vi "Tic Tac Toe.vi"() -> ()   [LabVIEW 2015]
panel:
  out "String 7":string="TIC TAC TOE GAME"
  in  "Tab Control":enum32{"Page 1", "Page 2"}(tab)
  in  "OK Button 9":bool
  in  "OK Button 8":bool
  in  "OK Button 7":bool
  in  "OK Button 6":bool
  in  "OK Button 5":bool
  in  "OK Button 4":bool
  in  "OK Button 3":bool
  in  "OK Button 2":bool
  in  "OK Button":bool
  in  "Text Colour X":u32(colorbox)
  in  "Text Colour O":u32(colorbox)
  in  "OK Button 12":bool
  in  "OK Button 11":bool
  out "Next Turn":string
  in  "OK Button 10":bool
  out "String 2":string="Player 1"
  out "String":string="Player 2"
  in  "Set Player Turn":bool
  out "String 6":string="O"
  out "String 5":string="X"
  out "String 10":string
  out "x .and. y?":bool
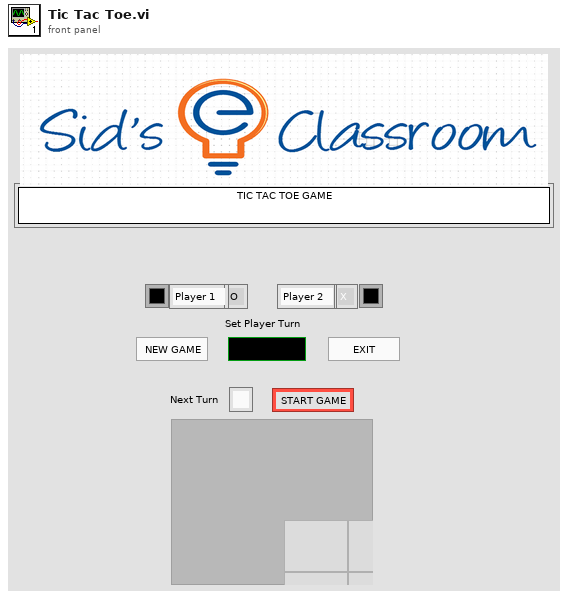
[diagram p1: front panel]
types:
  T1 = enum8{"Enabled", "Disabled", "Disabled and Grayed Out"}
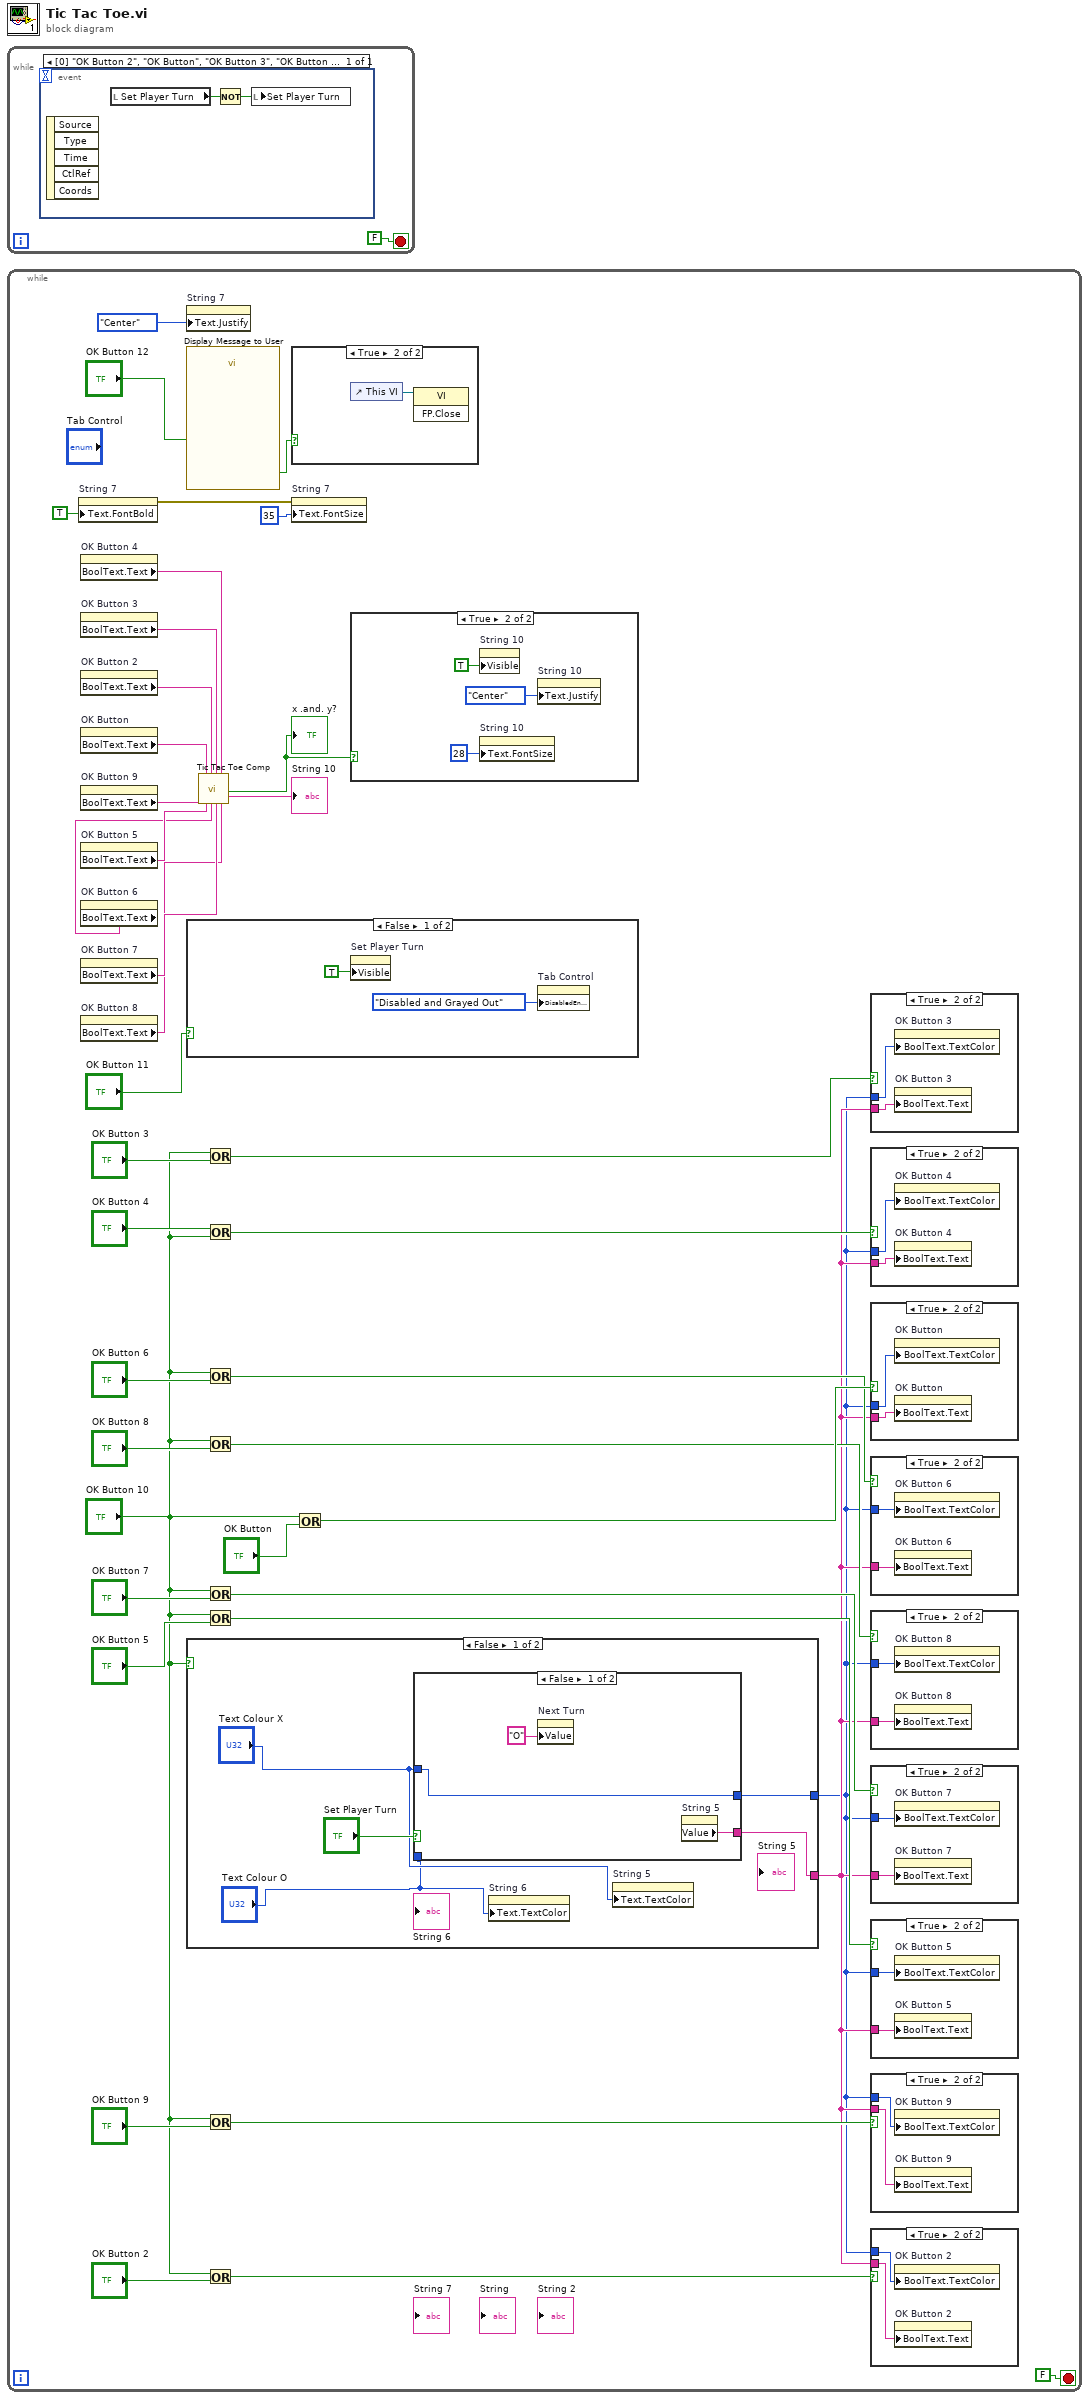
[diagram p0: block diagram]
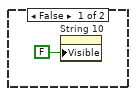
[diagram p2: hidden frame]
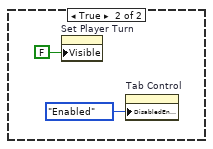
[diagram p4: hidden frame]
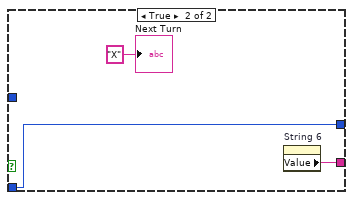
[diagram p5: hidden frame]
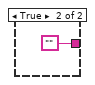
[diagram p6: hidden frame]
diagram:
  n1 = while {
    stop <- FALSE stop-if-true
    n2 = event shown="[0] \"OK Button 2\", \"OK Button\", \"OK Button 3\", \"OK Button 4\", \"OK Button 5\", \"OK Button 6\", \"OK Button 7\", \"OK Button 8\", \"OK Button 9\": Mouse Down" {
      selector: _ -> [_]
      dyn-events: _ -> [_]
      timeout: _ -> [_]
      event "OK Button 2", "OK Button", "OK Button 3", "OK Button 4", "OK Button 5", "OK Button 6", "OK Button 7", "OK Button 8", "OK Button 9": Mouse Down {
        n3 = event-data() -> ()  [unwired: 1 in, 5 out]
        n4 = local read "Set Player Turn"() -> (w3:bool)
        n5 = Not(x=w3) -> (.not. x?=w2:bool)
        n6 = local write "Set Player Turn"(w2) -> ()
      }
    }
  }
  n7 = while {
    stop <- FALSE stop-if-true
    n8 = property on="String 7" class="Str"("Text.FontBold"=TRUE ("Text.Font:Bold")) -> (error out=w6:errorcluster)  [unwired: 2 in, 1 out]
    n9 = property on="OK Button 4" class="Bool (strict)"() -> ("BoolText.Text"=w14:string)  [unwired: 2 in, 2 out]
    n10 = property on="OK Button 3" class="Bool (strict)"() -> ("BoolText.Text"=w15:string)  [unwired: 2 in, 2 out]
    n11 = property on="OK Button 2" class="Bool (strict)"() -> ("BoolText.Text"=w16:string)  [unwired: 2 in, 2 out]
    n12 = property on="OK Button" class="Bool (strict)"() -> ("BoolText.Text"=w17:string)  [unwired: 2 in, 2 out]
    n13 = property on="OK Button 9" class="Bool (strict)"() -> ("BoolText.Text"=w9:string)  [unwired: 2 in, 2 out]
    n14 = property on="OK Button 5" class="Bool (strict)"() -> ("BoolText.Text"=w13:string)  [unwired: 2 in, 2 out]
    n15 = property on="OK Button 6" class="Bool (strict)"() -> ("BoolText.Text"=w12:string)  [unwired: 2 in, 2 out]
    n16 = property on="OK Button 7" class="Bool (strict)"() -> ("BoolText.Text"=w11:string)  [unwired: 2 in, 2 out]
    n17 = property on="OK Button 8" class="Bool (strict)"() -> ("BoolText.Text"=w10:string)  [unwired: 2 in, 2 out]
    n18 = property on="String 7" class="Str"("Text.Justify"=enum16{"Left", "Center", "Right"}."Center" ("Text.Justification")) -> ()  [unwired: 2 in, 2 out]
    n19 = call "Display Message to User"("Enable"="OK Button 12") -> ("EXIT"=w20:bool)  [unwired: 9 in, 1 out]
    n20 = case shown="False" "OK Button 11" {
      frame False {
        n21 = property on="Set Player Turn" class="Bool (strict)"("Visible"=TRUE) -> ()  [unwired: 2 in, 2 out]
        n22 = property on="Tab Control" class="TabCtl (strict)"("DisabledEnum"=T1."Disabled and Grayed Out" ("Disabled")) -> ()  [unwired: 2 in, 2 out]
      }
      frame True {
        n23 = property on="Set Player Turn" class="Bool (strict)"("Visible"=FALSE) -> ()  [unwired: 2 in, 2 out]
        n24 = property on="Tab Control" class="TabCtl (strict)"("DisabledEnum"=T1."Enabled" ("Disabled")) -> ()  [unwired: 2 in, 2 out]
      }
    }
    n25 = case shown="False" "OK Button 10" {
      tunnel: [w56 ""] -> w23
      tunnel: [w55 _] -> w19
      frame False {
        n26 = case shown="False" "Set Player Turn" {
          tunnel: [w59 w62] -> w56
          tunnel: [w58 w61] -> w55
          tunnel: "Text Colour X" -> [w58 _]
          tunnel: "Text Colour O" -> [_ w61]
          frame False {
            n27 = property on="Next Turn" class="Str"("Value"="O" ("Current Symbol 2")) -> ()  [unwired: 2 in, 2 out]
            n28 = property on="String 5" class="Str"() -> ("Value"=w59:string)  [unwired: 2 in, 2 out]
          }
          frame True {
            n29 = property on="String 6" class="Str"() -> ("Value"=w62:string)  [unwired: 2 in, 2 out]
            "Next Turn" <- "X" ("Current Symbol")
          }
        }
        n30 = property on="String 6" class="Str"("Text.TextColor"="Text Colour O") -> ()  [unwired: 2 in, 2 out]
        n31 = property on="String 5" class="Str"("Text.TextColor"="Text Colour X") -> ()  [unwired: 2 in, 2 out]
      }
      frame True {
      }
    }
    n32 = call "Tic Tac Toe Comp.vi"("String 9"=w9, "String"=w17, "String 5"=w13, "String 2"=w16, "String 6"=w12, "String 3"=w15, "String 7"=w11, "String 4"=w14, "String 8"=w10) -> ("x .or. y?"=w8:bool, "String 10"=→"String 10":string)  [unwired: 9 in]
    "x .and. y?" <- w8
    n33 = Or(x="OK Button 10", y="OK Button 3") -> (x .or. y?=w25:bool)
    n34 = Or(x="OK Button 4", y="OK Button 10") -> (x .or. y?=w24:bool)
    n35 = Or(x="OK Button 10", y="OK Button 6") -> (x .or. y?=w37:bool)
    n36 = Or(x="OK Button 10", y="OK Button 8") -> (x .or. y?=w35:bool)
    n37 = Or(x="OK Button 10", y="OK Button 7") -> (x .or. y?=w33:bool)
    n38 = Or(x="OK Button 10", y="OK Button 5") -> (x .or. y?=w31:bool)
    n39 = Or(x="OK Button 10", y="OK Button 9") -> (x .or. y?=w29:bool)
    n40 = Or(x="OK Button 10", y="OK Button 2") -> (x .or. y?=w26:bool)
    n41 = case shown="True" w20 {
      frame False {
      }
      frame True {
        n42 = control-ref of="This VI"() -> (w48:refnum<vi>)
        n43 = invoke class="VI" method="FP.Close"(reference=w48) -> ()  [unwired: 2 in, 3 out]
      }
    }
    n44 = property on="String 7" class="Str"(error in=w6, "Text.FontSize"=u32 35 ("Text.Font:Size")) -> ()  [unwired: 1 in, 2 out]
    n45 = Or(x="OK Button 10", y="OK Button") -> (x .or. y?=w39:bool)
    n46 = case shown="True" w8 {
      frame False {
        n47 = property on="String 10" class="Str"("Visible"=FALSE) -> ()  [unwired: 2 in, 2 out]
      }
      frame True {
        n48 = property on="String 10" class="Str"("Visible"=TRUE) -> ()  [unwired: 2 in, 2 out]
        n49 = property on="String 10" class="Str"("Text.FontSize"=u32 28 ("Text.Font:Size")) -> ()  [unwired: 2 in, 2 out]
        n50 = property on="String 10" class="Str"("Text.Justify"=enum16{"Left", "Center", "Right"}."Center" ("Text.Justification")) -> ()  [unwired: 2 in, 2 out]
      }
    }
    n51 = case shown="True" w25 {
      tunnel: w23 -> [_ w68]
      tunnel: w19 -> [_ w67]
      frame False {
      }
      frame True {
        n52 = property on="OK Button 3" class="Bool (strict)"("BoolText.TextColor"=w67) -> ()  [unwired: 2 in, 2 out]
        n53 = property on="OK Button 3" class="Bool (strict)"("BoolText.Text"=w68) -> ()  [unwired: 2 in, 2 out]
      }
    }
    n54 = case shown="True" w24 {
      tunnel: w23 -> [_ w72]
      tunnel: w19 -> [_ w71]
      frame False {
      }
      frame True {
        n55 = property on="OK Button 4" class="Bool (strict)"("BoolText.TextColor"=w71) -> ()  [unwired: 2 in, 2 out]
        n56 = property on="OK Button 4" class="Bool (strict)"("BoolText.Text"=w72) -> ()  [unwired: 2 in, 2 out]
      }
    }
    n57 = case shown="True" w39 {
      tunnel: w23 -> [_ w82]
      tunnel: w19 -> [_ w81]
      frame False {
      }
      frame True {
        n58 = property on="OK Button" class="Bool (strict)"("BoolText.TextColor"=w81) -> ()  [unwired: 2 in, 2 out]
        n59 = property on="OK Button" class="Bool (strict)"("BoolText.Text"=w82) -> ()  [unwired: 2 in, 2 out]
      }
    }
    n60 = case shown="True" w37 {
      tunnel: w23 -> [_ w77]
      tunnel: w19 -> [_ w78]
      frame False {
      }
      frame True {
        n61 = property on="OK Button 6" class="Bool (strict)"("BoolText.TextColor"=w78) -> ()  [unwired: 2 in, 2 out]
        n62 = property on="OK Button 6" class="Bool (strict)"("BoolText.Text"=w77) -> ()  [unwired: 2 in, 2 out]
      }
    }
    n63 = case shown="True" w35 {
      tunnel: w23 -> [_ w76]
      tunnel: w19 -> [_ w75]
      frame False {
      }
      frame True {
        n64 = property on="OK Button 8" class="Bool (strict)"("BoolText.TextColor"=w75) -> ()  [unwired: 2 in, 2 out]
        n65 = property on="OK Button 8" class="Bool (strict)"("BoolText.Text"=w76) -> ()  [unwired: 2 in, 2 out]
      }
    }
    n66 = case shown="True" w33 {
      tunnel: w23 -> [_ w74]
      tunnel: w19 -> [_ w73]
      frame False {
      }
      frame True {
        n67 = property on="OK Button 7" class="Bool (strict)"("BoolText.TextColor"=w73) -> ()  [unwired: 2 in, 2 out]
        n68 = property on="OK Button 7" class="Bool (strict)"("BoolText.Text"=w74) -> ()  [unwired: 2 in, 2 out]
      }
    }
    n69 = case shown="True" w31 {
      tunnel: w23 -> [_ w66]
      tunnel: w19 -> [_ w65]
      frame False {
      }
      frame True {
        n70 = property on="OK Button 5" class="Bool (strict)"("BoolText.TextColor"=w65) -> ()  [unwired: 2 in, 2 out]
        n71 = property on="OK Button 5" class="Bool (strict)"("BoolText.Text"=w66) -> ()  [unwired: 2 in, 2 out]
      }
    }
    n72 = case shown="True" w29 {
      tunnel: w23 -> [_ w80]
      tunnel: w19 -> [_ w79]
      frame False {
      }
      frame True {
        n73 = property on="OK Button 9" class="Bool (strict)"("BoolText.TextColor"=w79) -> ()  [unwired: 2 in, 2 out]
        n74 = property on="OK Button 9" class="Bool (strict)"("BoolText.Text"=w80) -> ()  [unwired: 2 in, 2 out]
      }
    }
    n75 = case shown="True" w26 {
      tunnel: w23 -> [_ w70]
      tunnel: w19 -> [_ w69]
      frame False {
      }
      frame True {
        n76 = property on="OK Button 2" class="Bool (strict)"("BoolText.TextColor"=w69) -> ()  [unwired: 2 in, 2 out]
        n77 = property on="OK Button 2" class="Bool (strict)"("BoolText.Text"=w70) -> ()  [unwired: 2 in, 2 out]
      }
    }
  }
